vi "subEventLoopForStatus.vi"(8 "error in (no error)":errorcluster, 9 "Events":T1, 11 "MulticolumnListbox in":refnum<vi>) -> (0 "error out":errorcluster)   [LabVIEW 2020, in "SolutionBuilder.lvlib"]
uses:
  SolutionBuilder/SolutionBuilder.lvlib
  SolutionBuilder/Events.ctl
  SolutionBuilder/EventUpdateList.ctl
  SolutionBuilder/EventItemBuilt.ctl
  SolutionBuilder/SolutionBuilder.lvclass
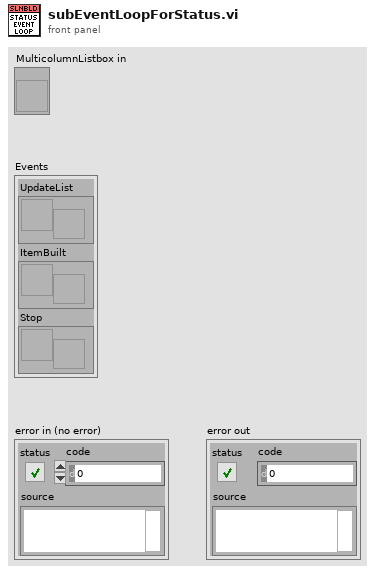
[diagram p1: front panel]
types:
  T1 = typedef "SolutionBuilder.lvlib/Events.ctl" = cluster{"UpdateList":T2, "ItemBuilt":T3, "Stop":refnum<user-event>}
  T2 = typedef "SolutionBuilder.lvlib/SolutionBuilder.lvclass/EventUpdateList.ctl" = refnum<user-event>
  T3 = typedef "SolutionBuilder.lvlib/SolutionBuilder.lvclass/EventItemBuilt.ctl" = refnum<user-event>
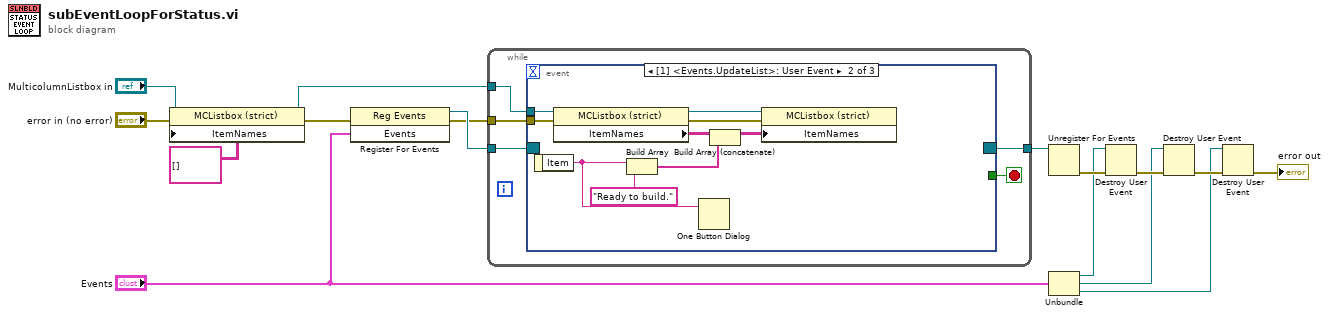
[diagram p0: block diagram]
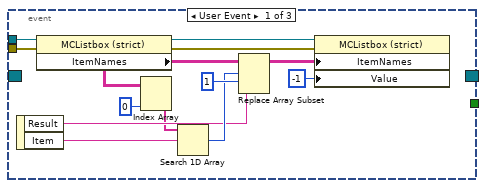
[diagram p2: hidden frame]
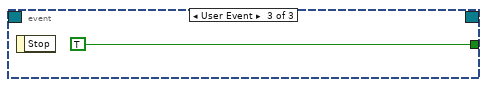
[diagram p3: hidden frame]
diagram:
  n1 = property class="MCListbox (strict)"(reference="MulticolumnListbox in", error in="error in (no error)", "ItemNames"=string[][] [] ("Item Names")) -> (reference out=w5:refnum<vi>, error out=w7:errorcluster)
  n2 = register-events(error in=w7, "Events") -> (reference out=w13:refnum<event-registration>, error out=w12:errorcluster)  [unwired: 1 in]
  n3 = while {
    tunnel: w12 -> [w21]
    tunnel: w13 -> [w20]
    tunnel: w5 -> [w18]
    tunnel: [w17] -> w14
    stop <- w19 stop-if-true
    n4 = event shown="[1] <Events.UpdateList>: User Event" {
      selector: w20 -> [_ _ _]
      dyn-events: [_ _ _] -> w17
      timeout: _ -> [_ _ _]
      tunnel: w21 -> [w31 w43 _]
      tunnel: [_ _ TRUE] -> w19
      tunnel: w18 -> [w32 w42 _]
      event User Event {
        n5 = event-data() -> ("Result"=w26:string, "Item"=w27:string)  [unwired: 1 in]
        n6 = property class="MCListbox (strict)"(reference=w32, error in=w31) -> (reference out=w30:refnum<vi>, error out=w29:errorcluster, "ItemNames"=w25:string[][])
        n7 = Index Array(array=w25, index (col)=0 ("disabled index (col)")) -> (element=w23:string[])  [unwired: 1 in]
        n8 = Search 1D Array(1D array=w23, element=w27) -> (index of element=w33:i32)  [unwired: 1 in]
        n9 = Replace Array Subset(array=w25, new element=w26, index (row)=w33, index (col)=1 ("disabled index (col)")) -> (w28:string[][])
        n10 = property class="MCListbox (strict)"(reference=w30, error in=w29, "ItemNames"=w28, "Value"=-1) -> ()  [unwired: 2 out]
      }
      event User Event {
        n11 = event-data() -> ("Item"=w35:string)  [unwired: 1 in]
        n12 = property class="MCListbox (strict)"(reference=w42, error in=w43) -> (reference out=w36:refnum<vi>, error out=w37:errorcluster, "ItemNames"=w41:string[][])
        n13 = Build Array(w35, "Ready to build." ("element")) -> (w39:string[])
        n14 = One Button Dialog(message=w35) -> ()  [unwired: 1 in, 1 out]
        n15 = Build Array (concatenate)(w41, w39) -> (w38:string[][])
        n16 = property class="MCListbox (strict)"(reference=w36, error in=w37, "ItemNames"=w38) -> ()  [unwired: 2 out]
      }
      event User Event {
        n17 = event-data() -> ()  [unwired: 1 in, 1 out]
      }
    }
  }
  n18 = Unregister For Events(event registration refnum=w14) -> (error out=w15:errorcluster)  [unwired: 1 in]
  n19 = Unbundle("Events") -> ("UpdateList"=w2:T2, "ItemBuilt"=w1:T3, "Stop"=w3:refnum<user-event>)
  n20 = Destroy User Event(user event=w2, error in=w15) -> (error out=w16:errorcluster)
  n21 = Destroy User Event(user event=w1, error in=w16) -> (error out=w11:errorcluster)
  n22 = Destroy User Event(user event=w3, error in=w11) -> (error out=→"error out":errorcluster)
